vi "Front Panel to Parameters.vi"(8 "error in (no error)":errorcluster, 11 "RUS Measurement in":refnum<class "RUS Measurement.lvclass">) -> (0 "error out":errorcluster, 3 "RUS Measurement out":refnum<class "RUS Measurement.lvclass">)   [LabVIEW 2015, in "RUS Measurement.lvclass"]
uses:
  RUS Measurement.lvclass
  RUS Measurement.lvclass/RUS Measurement.ctl
  Mag Lab Measurement/Mag Lab Measurement.lvclass
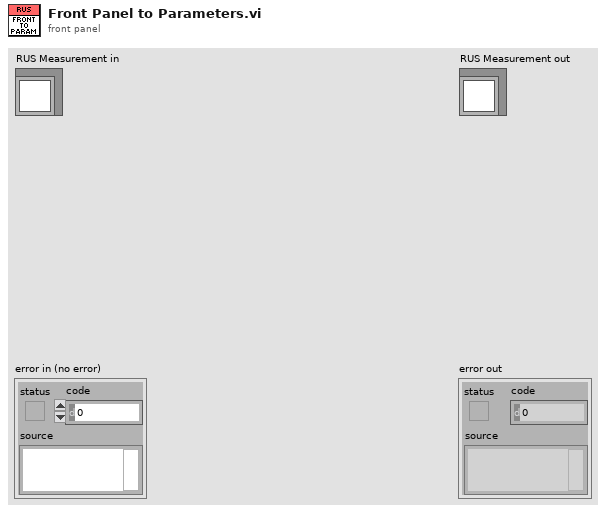
[diagram p1: front panel]
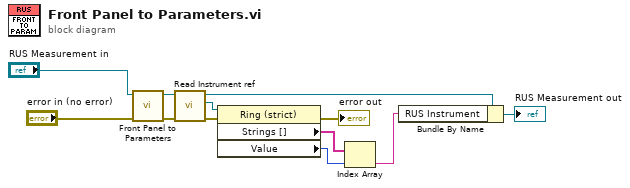
[diagram p0: block diagram]
diagram:
  n1 = call-parent "Front Panel to Parameters.vi"("error in (no error)"="error in (no error)", "Mag Lab Root in"="RUS Measurement in") -> ("error out"=w4:errorcluster, "Mag Lab Root out"=w12:refnum<class "RUS Measurement.lvclass">)  [unwired: 8 in]
  n2 = call "Read Instrument ref.vi"("error in (no error)"=w4, "RUS Measurement in"=w12) -> ("error out"=w5:errorcluster, "Instrument ref"=w8:refnum<vi>, "RUS Measurement out"=w9:refnum<class "RUS Measurement.lvclass">)  [unwired: 7 in]
  n3 = property class="Ring (strict)"(reference=w8, error in=w5) -> (error out=→"error out":errorcluster, "Strings []"=w7:string[], "Value"=w6:u16)  [unwired: 1 out]
  n4 = Index Array(array=w7, index=w6) -> (element=w2:string)
  n5 = Bundle By Name(cluster=w9, "RUS Instrument"=w2) -> (→"RUS Measurement out":refnum<class "RUS Measurement.lvclass">)
